vi "RT_mem_i6(SubVI).vi"(8 "Ini_val":dbl, 10 "start":bool, 11 "In":dbl format="%#_13g") -> (1 "in_vec":dbl[](array[numeric]), 3 "in_i6":dbl)   [LabVIEW 2017]
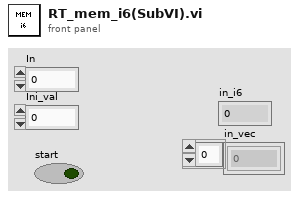
[diagram p1: front panel]
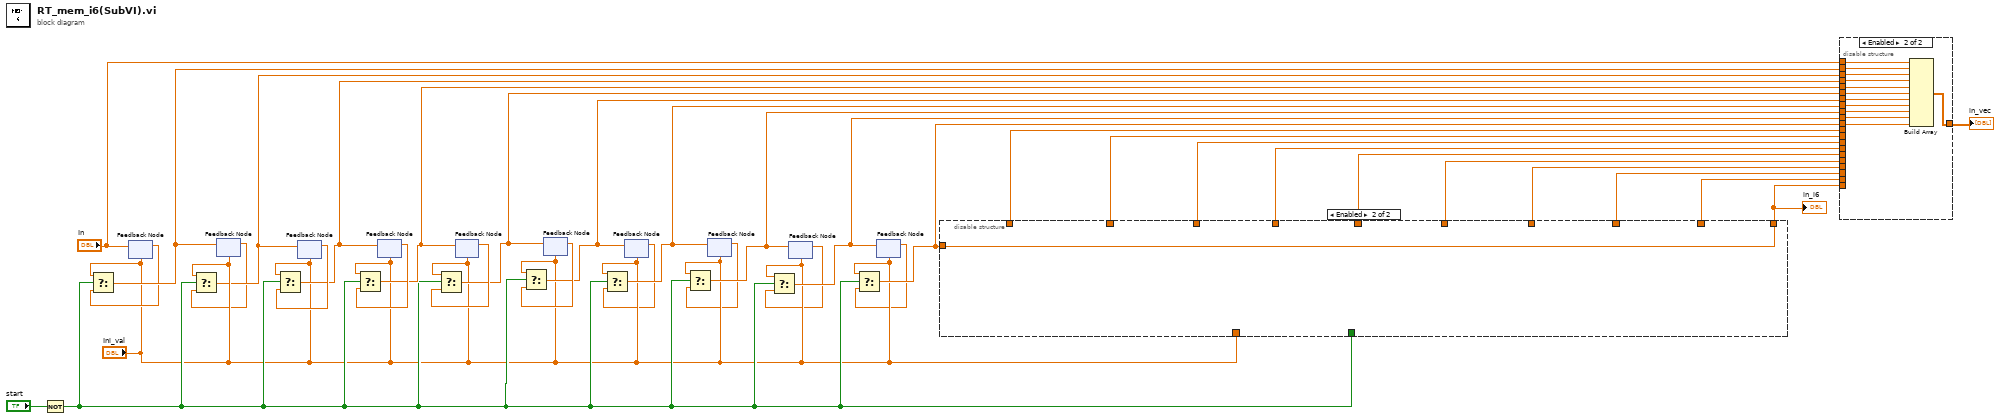
[diagram p0: block diagram]
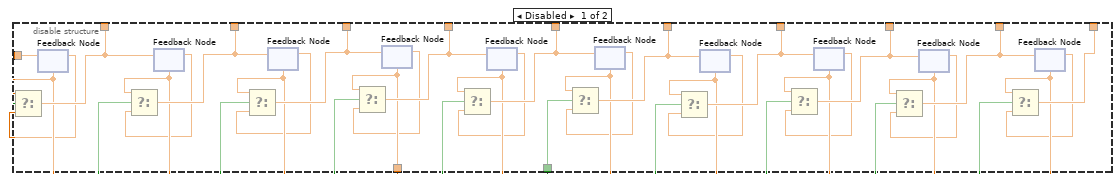
[diagram p2: hidden frame]
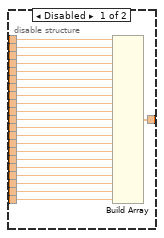
[diagram p3: hidden frame]
diagram:
  n1 = Not(x="start") -> (.not. x?=w8:bool)
  n2 = feedback #1("Ini_val") -> (w9:dbl)
  n3 = Select(t="Ini_val", s=w8, f=w9) -> (s? t:f=w10:dbl)
  n4 = feedback-in #1("In") -> ()
  n5 = feedback #2("Ini_val") -> (w5:dbl)
  n6 = Select(t="Ini_val", s=w8, f=w5) -> (s? t:f=w6:dbl)
  n7 = feedback-in #2(w10) -> ()
  n8 = feedback #3("Ini_val") -> (w32:dbl)
  n9 = Select(t="Ini_val", s=w8, f=w32) -> (s? t:f=w31:dbl)
  n10 = feedback-in #3(w6) -> ()
  n11 = feedback #4("Ini_val") -> (w33:dbl)
  n12 = Select(t="Ini_val", s=w8, f=w33) -> (s? t:f=w30:dbl)
  n13 = feedback-in #4(w31) -> ()
  n14 = feedback #5("Ini_val") -> (w34:dbl)
  n15 = Select(t="Ini_val", s=w8, f=w34) -> (s? t:f=w29:dbl)
  n16 = feedback-in #5(w30) -> ()
  n17 = feedback #6("Ini_val") -> (w35:dbl)
  n18 = Select(t="Ini_val", s=w8, f=w35) -> (s? t:f=w28:dbl)
  n19 = feedback-in #6(w29) -> ()
  n20 = feedback #7("Ini_val") -> (w2:dbl)
  n21 = Select(t="Ini_val", s=w8, f=w2) -> (s? t:f=w27:dbl)
  n22 = feedback-in #7(w28) -> ()
  n23 = feedback #8("Ini_val") -> (w1:dbl)
  n24 = Select(t="Ini_val", s=w8, f=w1) -> (s? t:f=w26:dbl)
  n25 = feedback-in #8(w27) -> ()
  n26 = feedback #9("Ini_val") -> (w4:dbl)
  n27 = Select(t="Ini_val", s=w8, f=w4) -> (s? t:f=w25:dbl)
  n28 = feedback-in #9(w26) -> ()
  n29 = feedback #10("Ini_val") -> (w3:dbl)
  n30 = Select(t="Ini_val", s=w8, f=w3) -> (s? t:f=w24:dbl)
  n31 = feedback-in #10(w25) -> ()
  n32 = disable-structure shown="Enabled" {
    disable-tunnel: w24 -> [w58 w59]
    disable-tunnel: [w57 _] -> w23
    disable-tunnel: [w56 _] -> w22
    disable-tunnel: [w55 _] -> w21
    disable-tunnel: [w54 _] -> w20
    disable-tunnel: [w53 _] -> w19
    disable-tunnel: [w52 _] -> w18
    disable-tunnel: [w51 _] -> w17
    disable-tunnel: [w50 _] -> w16
    disable-tunnel: [w49 _] -> w15
    disable-tunnel: [w48 w59] -> w14
    disable-tunnel: w8 -> [w47 _]
    disable-tunnel: "Ini_val" -> [w46 _]
    frame Disabled {
      n33 = feedback #11(w46) -> (w36:dbl)
      n34 = Select(t=w46, s=w47, f=w36) -> (s? t:f=w57:dbl)
      n35 = feedback-in #11(w58) -> ()
      n36 = feedback #12(w46) -> (w37:dbl)
      n37 = Select(t=w46, s=w47, f=w37) -> (s? t:f=w56:dbl)
      n38 = feedback-in #12(w57) -> ()
      n39 = feedback #13(w46) -> (w45:dbl)
      n40 = Select(t=w46, s=w47, f=w45) -> (s? t:f=w55:dbl)
      n41 = feedback-in #13(w56) -> ()
      n42 = feedback #14(w46) -> (w42:dbl)
      n43 = Select(t=w46, s=w47, f=w42) -> (s? t:f=w54:dbl)
      n44 = feedback-in #14(w55) -> ()
      n45 = feedback #15(w46) -> (w43:dbl)
      n46 = Select(t=w46, s=w47, f=w43) -> (s? t:f=w53:dbl)
      n47 = feedback-in #15(w54) -> ()
      n48 = feedback #16(w46) -> (w44:dbl)
      n49 = Select(t=w46, s=w47, f=w44) -> (s? t:f=w52:dbl)
      n50 = feedback-in #16(w53) -> ()
      n51 = feedback #17(w46) -> (w38:dbl)
      n52 = Select(t=w46, s=w47, f=w38) -> (s? t:f=w51:dbl)
      n53 = feedback-in #17(w52) -> ()
      n54 = feedback #18(w46) -> (w41:dbl)
      n55 = Select(t=w46, s=w47, f=w41) -> (s? t:f=w50:dbl)
      n56 = feedback-in #18(w51) -> ()
      n57 = feedback #19(w46) -> (w40:dbl)
      n58 = Select(t=w46, s=w47, f=w40) -> (s? t:f=w49:dbl)
      n59 = feedback-in #19(w50) -> ()
      n60 = feedback #20(w46) -> (w39:dbl)
      n61 = Select(t=w46, s=w47, f=w39) -> (s? t:f=w48:dbl)
      n62 = feedback-in #20(w49) -> ()
    }
    frame Enabled {
    }
  }
  "in_i6" <- w14
  n63 = disable-structure shown="Enabled" {
    disable-tunnel: w31 -> [w81 w90]
    disable-tunnel: w30 -> [w80 w89]
    disable-tunnel: w29 -> [w79 w88]
    disable-tunnel: w28 -> [w78 w87]
    disable-tunnel: w27 -> [w77 w85]
    disable-tunnel: w26 -> [w76 w84]
    disable-tunnel: w25 -> [w75 w83]
    disable-tunnel: w24 -> [w74 w82]
    disable-tunnel: w23 -> [w73 _]
    disable-tunnel: w22 -> [w72 _]
    disable-tunnel: w21 -> [w71 _]
    disable-tunnel: w20 -> [w70 _]
    disable-tunnel: w19 -> [w69 _]
    disable-tunnel: w18 -> [w68 _]
    disable-tunnel: w17 -> [w67 _]
    disable-tunnel: w16 -> [w66 _]
    disable-tunnel: w15 -> [w65 _]
    disable-tunnel: w14 -> [w64 _]
    disable-tunnel: [w63 w86] -> w13
    disable-tunnel: "In" -> [w62 w93]
    disable-tunnel: w10 -> [w61 w92]
    disable-tunnel: w6 -> [w60 w91]
    frame Disabled {
      n64 = Build Array(w62, w61, w60, w81, w80, w79, w78, w77, w76, w75, w74, w73, w72, w71, w70, w69, w68, w67, w66, w65, w64) -> (w63:dbl[])
    }
    frame Enabled {
      n65 = Build Array(w93, w92, w91, w90, w89, w88, w87, w85, w84, w83, w82) -> (w86:dbl[])
    }
  }
  "in_vec" <- w13
